vi "ANAL_DataGrapher.vi"(5 "Software Gate":cluster{"Numeric":i32, "Numeric":i32}(slide)={"Numeric"=96, "Numeric"=937} scale=0.0..1023.0, 7 "Sweep Range":cluster{"Numeric":i32, "Numeric":i32}(slide)={"Numeric"=0, "Numeric"=4} scale=0.0..10.0, 9 "GUI Cluster":T6, 10 "Main Data Array":T3 {"Run Data Cluster"."Temperature B" scale=0.0..100.0; "Run Data Cluster"."Temperature A" scale=0.0..100.0}, 11 "AorB":bool) -> (0 "Time Array":T2(array[cluster]), 1 "Bin Graph":cluster{"Numeric":i32, "element":i32}[](array[cluster]), 2 "Main Data Array Out":T3 {"Run Data Cluster"."Temperature B" scale=0.0..100.0; "Run Data Cluster"."Temperature A" scale=0.0..100.0}, 4 "Temp Array":T1(array[cluster]))   [LabVIEW 2021]
uses:
  ANAL_Data.ctl
  XML_Cluster.ctl
  DAT_Cluster.ctl
  ANAL_GUIStatus.ctl
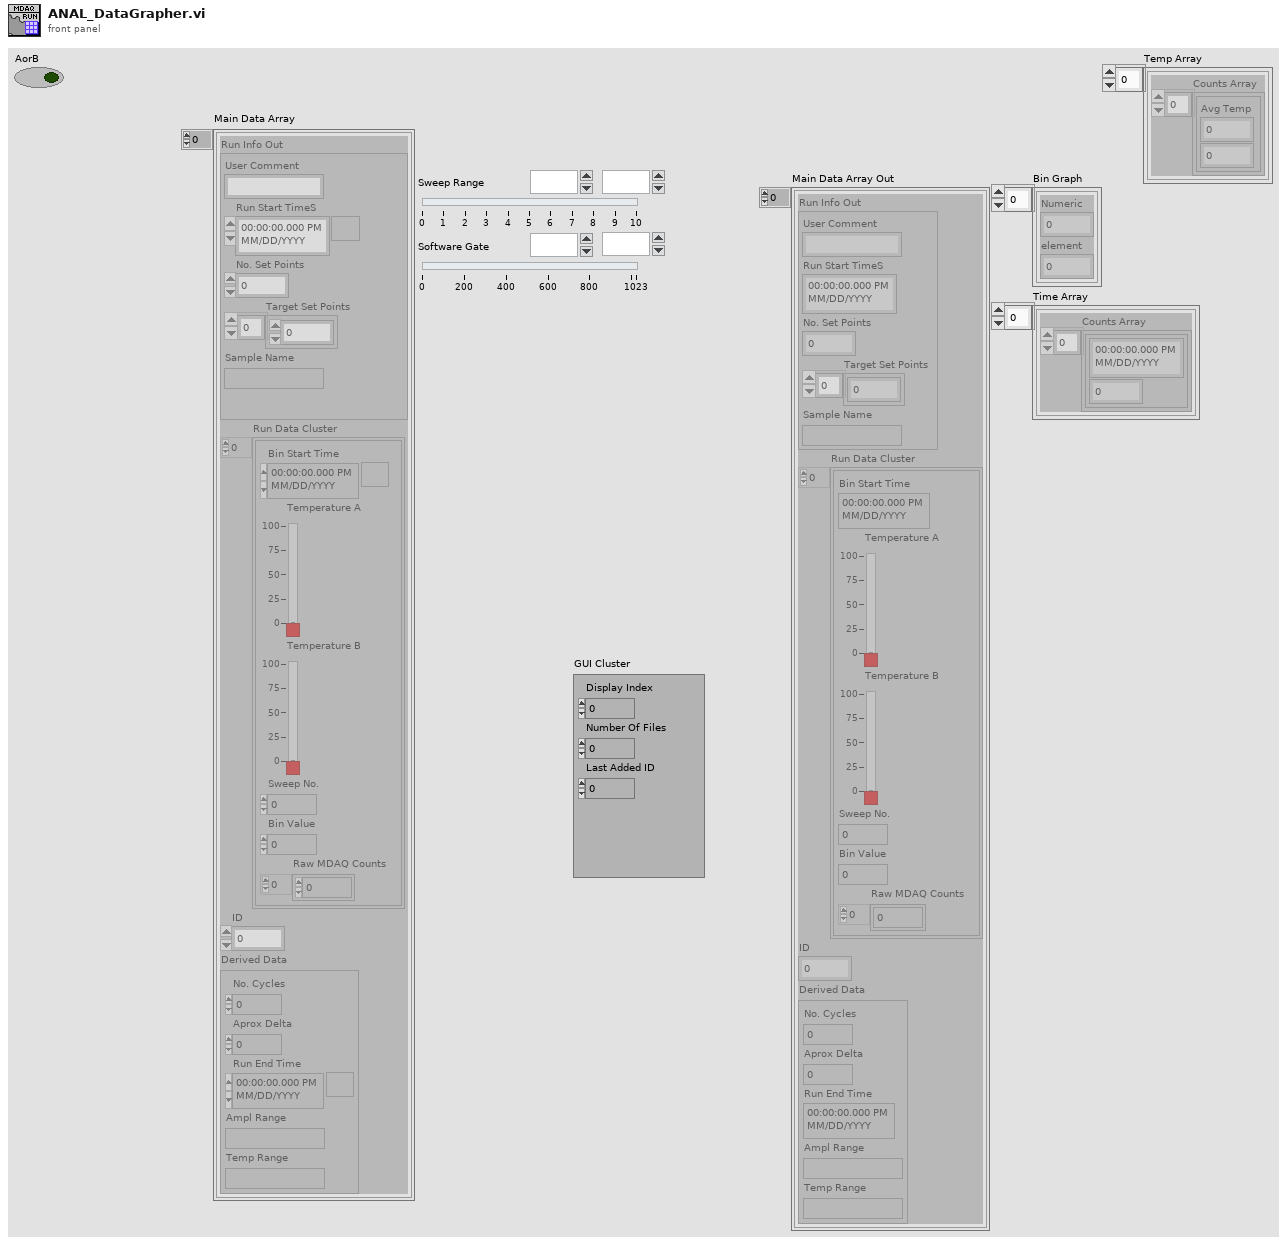
[diagram p1: front panel]
types:
  T1 = cluster{"Counts Array":cluster{"Avg Temp":dbl, i32}[]}[]
  T2 = cluster{"Counts Array":cluster{timestamp, dbl}[]}[]
  T3 = typedef "ANAL_Data.ctl" = cluster{"Run Info Out":T4, "Run Data Cluster":T5, "ID":u32, "Derived Data":cluster{"No. Cycles":u32, "Aprox Delta":dbl, "Run End Time":timestamp, "Ampl Range":string, "Temp Range":string}}[]
  T4 = typedef "XML_Cluster.ctl" = cluster{"User Comment":string, "Run Start TimeS":timestamp, "No. Set Points":u32, "Target Set Points":i32[], "Sample Name":string}
  T5 = typedef "DAT_Cluster.ctl" = cluster{"Bin Start Time":timestamp, "Temperature A":dbl, "Temperature B":dbl, "Sweep No.":i32, "Bin Value":i32, "Raw MDAQ Counts":i32[]}[]
  T6 = typedef "ANAL_GUIStatus.ctl" = cluster{"Display Index":i32, "Number Of Files":u32, "Last Added ID":u32}
  T7 = cluster{"Run Info Out":T4, "Run Data Cluster":T5, "ID":u32, "Derived Data":cluster{"No. Cycles":u32, "Aprox Delta":dbl, "Run End Time":timestamp, "Ampl Range":string, "Temp Range":string}}
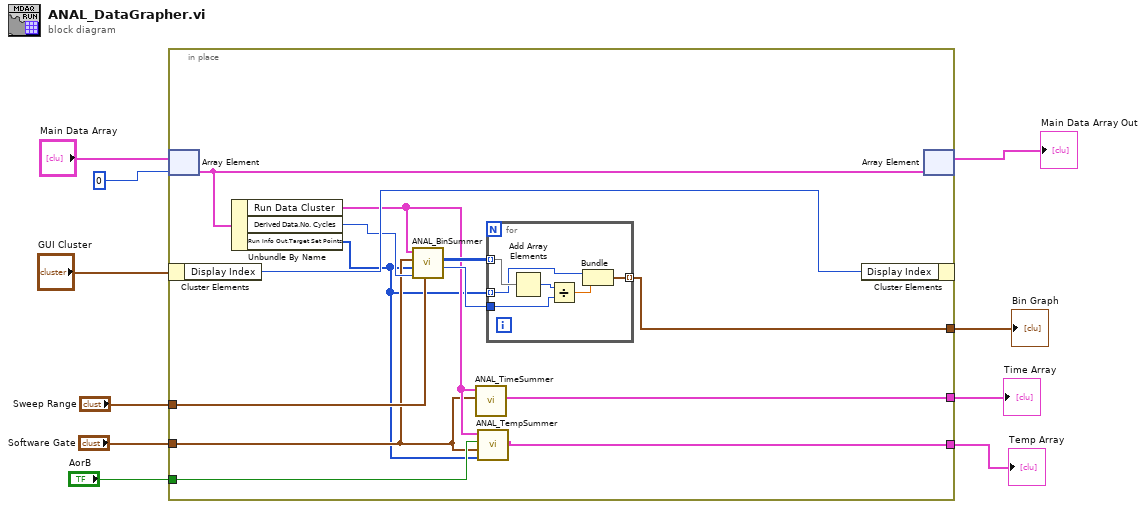
[diagram p0: block diagram]
diagram:
  n1 = in-place {
    in-place-border: "Sweep Range" -> [w22]
    in-place-border: "Software Gate" -> [w13]
    in-place-border: [w18] -> w4
    in-place-border: [w16] -> w3
    in-place-border: "AorB" -> [w14]
    in-place-border: [w11] -> w1
    n2 = in-place-array #1("Main Data Array", 0) -> (w23:T7)
    n3 = in-place-cluster #2("GUI Cluster") -> ("Display Index"=w21:i32)
    n4 = Unbundle By Name(w23) -> ("Run Data Cluster"=w15:T5, "Derived Data.No. Cycles"=w20:u32, "Run Info Out.Target Set Points"=w12:i32[])
    n5 = call "ANAL_BinSummer.vi"("Sweep Range"=w22, "No. Cycles"=w20, "Target Set Points"=w12, "Software Gate"=w13, "Run Data Cluster"=w15) -> ("Sweeps"=w17:i32, "PackedArray"=w19:i32[][])  [unwired: 5 in]
    n6 = call "ANAL_TimeSummer.vi"("Software Gate"=w13, "Run Data Cluster"=w15) -> ("Time Array"=w16:T2)  [unwired: 9 in]
    n7 = call "ANAL_TempSummer.vi"("Target Set Points"=w12, "Software Gate"=w13, "AorB"=w14, "Run Data Cluster"=w15) -> ("Temp Array"=w11:T1)  [unwired: 7 in]
    n8 = for {
      tunnel: w19 -> [w29] mode=indexing
      tunnel: w12 -> [w28] mode=indexing
      tunnel: [w27] -> w18 mode=indexing
      tunnel: w17 -> [w24]
      n9 = Add Array Elements(numeric array=w29) -> (sum=w25:i32)
      n10 = Divide(x=w25, y=w24) -> (x/y=w26:dbl)
      n11 = Bundle("Numeric"=w28, w26) -> (w27:cluster{"Numeric":i32, dbl})  [unwired: 1 in]
    }
    n12 = in-place-cluster #2("Display Index"=w21) -> ()  [unwired: 1 out]
    n13 = in-place-array #1(w23) -> (→"Main Data Array Out":T3)  [unwired: 1 out]
  }
  "Bin Graph" <- w4
  "Time Array" <- w3
  "Temp Array" <- w1
